vi "AnalogWaveformProbe_CSG_mag.vi"(1 "Waveform":waveform(csg)={"t0"=timestamp(0 s since 1904-01-01), "dt"=0.0, "Y"=[]}) -> (0 "Stop if?":bool)   [LabVIEW 2017]
doc: "Displays a graph of the analog data; a table with a time stamp that specifies when the probe received the data, the x value, and the time; and a table that displays the attributes of the waveform data type."
uses:
  <vilib>/Utility/error.llb/ErrWarn.ctl
panel:
  in  "x":string="x"
  in  "t":string="t"
  in  "Tab Control":T1(tab)
  out "Timestamp":timestamp format="%<%X\n%x>T"
  out "Waveform Graph":waveform(dbl)(graph) caption="Waveform Graph 2"
  in  "warn icon":T2
  in  "warning msg":string="Table data truncated to\nlimit memory usage."
  out "Start t":timestamp format="%<%X\n%x>T"
  out "Data":string[][](table)
  out "Attributes":variant
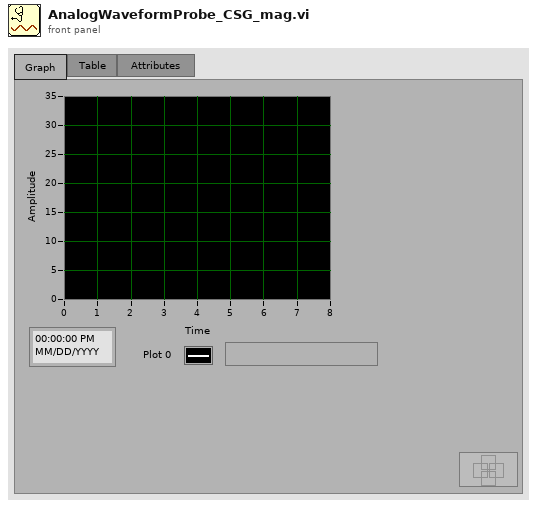
[diagram p1: front panel]
types:
  T1 = enum32{"Graph   ", "Table   ", "Attributes     "}
  T2 = typedef "ErrWarn.ctl" = bool
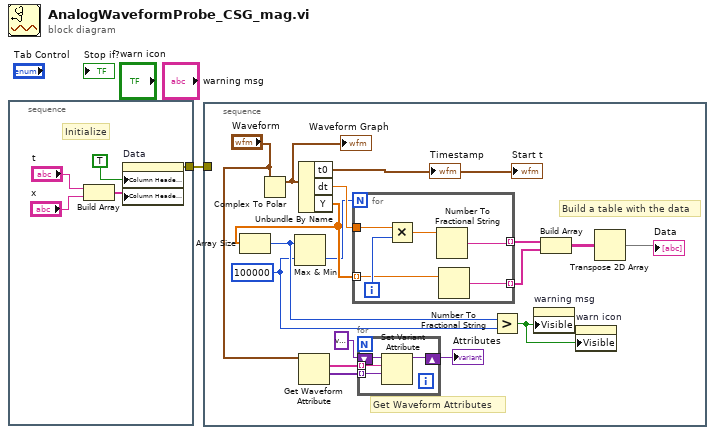
[diagram p0: block diagram]
diagram:
  n1 = stacked-sequence {
    tunnel: [w2] -> w1
    frame #0 {
      # "Initialize"
      n2 = Build Array("t", "x") -> (w4:string[])
      n3 = property on="Data" class="Tbl (strict)"("Column Headers Visible"=TRUE, "Column Header Strings[]"=w4) -> (error out=w2:errorcluster)  [unwired: 2 in, 1 out]
    }
  }
  n4 = stacked-sequence {
    tunnel: w1 -> [_]
    frame #0 {
      w10 = 100000
      # "Get Waveform Attributes"
      # "Build a table with the data"
      n5 = Complex To Polar(r * e^(i*theta)="Waveform") -> (r=w7:waveform(dbl))  [unwired: 1 out]
      "Waveform Graph" <- w7
      n6 = Unbundle By Name(w7) -> ("t0"=→"Timestamp" →"Start t":timestamp, "dt"=w23:dbl, "Y"=w13:dbl[])
      n7 = Array Size(array=w13) -> (size(s)=w11:i32)
      n8 = Max & Min(x=w11, y=w10) -> (min(x,y)=w12:i32)  [unwired: 1 out]
      n9 = Get Waveform Attribute(7:"Waveform") -> (1:w16:variant[], 2:w17:string[])  [unwired: 3 in, 2 out]
      n10 = for {
        N: w12 -> [_]
        tunnel: [w31] -> w20 mode=indexing
        tunnel: w13 -> [w30] mode=indexing
        tunnel: w23 -> [w33]
        tunnel: [w28] -> w19 mode=indexing
        i -> [w32]
        n11 = Multiply(x=w33, y=w32) -> (x*y=w29:dbl)
        n12 = Number To Fractional String(number=w29) -> (F-format string=w28:string)  [unwired: 3 in]
        n13 = Number To Fractional String(number=w30) -> (F-format string=w31:string)  [unwired: 3 in]
      }
      n14 = for {
        tunnel: w17 -> [w26] mode=indexing
        tunnel: w16 -> [w27] mode=indexing
        shift-right: [w24] -> w14
        shift-left: variant ("variant") -> [w25]
        n15 = Set Variant Attribute(Variant=w25, name=w26, value=w27) -> (Variant out=w24:variant)  [unwired: 1 in, 2 out]
      }
      "Attributes" <- w14
      n16 = Greater?(x=w11, y=w10) -> (0:w9:bool)
      n17 = property on="warning msg" class="Str"("Visible"=w9) -> ()  [unwired: 2 in, 2 out]
      n18 = Build Array(w19, w20) -> (w22:string[][])
      n19 = property on="warn icon" class="Bool"("Visible"=w9) -> ()  [unwired: 2 in, 2 out]
      n20 = Transpose 2D Array(2D array=w22) -> (transposed array=→"Data":string[][])
    }
  }
